vi "ScaleAllValue.vi"(0 "properties":T2[](array[typedef]), 1 "Caps":T1, 5 "error in (no error)":errorcluster, 6 "physical channel":string) -> (14 "Init Value":variant[](array[variant]), 19 "error out":errorcluster)   [LabVIEW 2018]
uses:
  Ctrl/Property.ctl
  Ctrl/Caps.ctl
  Ctrl/PhysicalChannel.ctl
  Ctrl/Register.ctl
  Ctrl/Bitfield.ctl
  Ctrl/Scale.ctl
  Ctrl/ScaleType.ctl
  Ctrl/Enum.ctl
  Ctrl/EnumValue.ctl
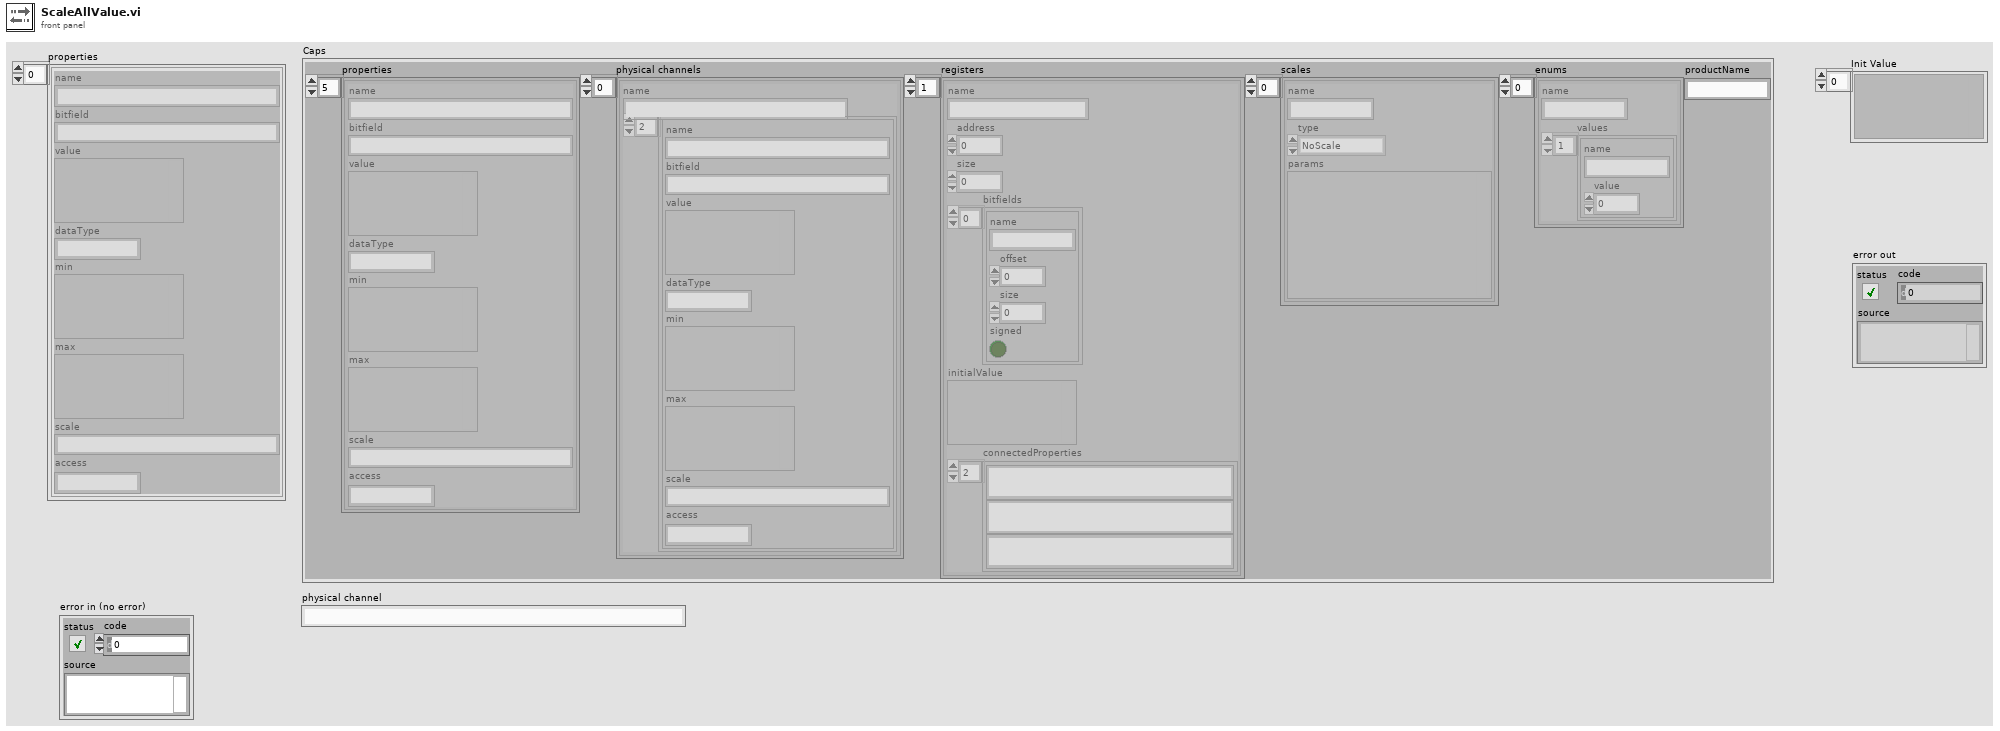
[diagram p1: front panel]
types:
  T1 = typedef "Caps.ctl" = cluster{"properties":T2[], "physical channels":T3[], "registers":T4[], "scales":T6[], "enums":T8[], "productName":string}
  T2 = typedef "Property.ctl" = cluster{"name":string, "bitfield":string, "value":variant, "dataType":string, "min":variant, "max":variant, "scale":string, "access":string}
  T3 = typedef "PhysicalChannel.ctl" = cluster{"name":string, "properties":T2[]}
  T4 = typedef "Register.ctl" = cluster{"name":string, "address":i32, "size":i32, "bitfields":T5[], "initialValue":variant, "connectedProperties":string[]}
  T5 = typedef "Bitfield.ctl" = cluster{"name":string, "offset":i32, "size":i32, "signed":bool}
  T6 = typedef "Scale.ctl" = cluster{"name":string, "type":T7, "params":variant}
  T7 = typedef "ScaleType.ctl" = enum16{"NoScale", "Table", "Polynomial", "Linear"}
  T8 = typedef "Enum.ctl" = cluster{"name":string, "values":T9[]}
  T9 = typedef "EnumValue.ctl" = cluster{"name":string, "value":i32}
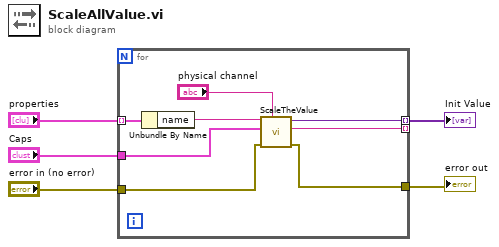
[diagram p0: block diagram]
diagram:
  n1 = for {
    tunnel: [w13] -> w1 mode=indexing
    tunnel: "properties" -> [w12] mode=indexing
    tunnel: "Caps" -> [w10]
    tunnel: "error in (no error)" -> [w9]
    tunnel: [w8] -> w2
    tunnel: [w6] -> _ mode=indexing
    n2 = Unbundle By Name(w12) -> ("name"=w11:string)
    n3 = call "ScaleTheValue.vi"("physical channel"="physical channel", "error in (no error)"=w9, "Caps"=w10, "property"=w11) -> ("error out"=w8:errorcluster, "dataType"=w6:string, "offline value"=w13:variant)  [unwired: 5 in]
  }
  "Init Value" <- w1
  "error out" <- w2
